vi "Client References Find Reference.vi"(2 "ID to Find (\"\")":string, 3 "TESTREFS (empty)":T1[](array[typedef])) -> (1 "Element":i32)   [LabVIEW 2011]
uses:
  Client References.ctl
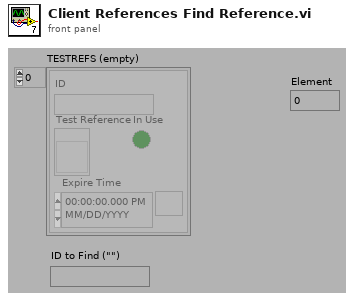
[diagram p1: front panel]
types:
  T1 = typedef "Client References.ctl" = cluster{"ID":string, "Test Reference":refnum<vi>, "In Use":bool, "Expire Time":timestamp}
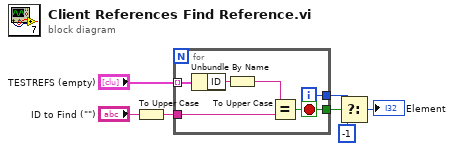
[diagram p0: block diagram]
diagram:
  n1 = To Upper Case(1:"ID to Find (\"\")") -> (0:w7:string)
  n2 = for {
    tunnel: "TESTREFS (empty)" -> [w13] mode=indexing
    tunnel: w7 -> [w12]
    tunnel: [w10] -> w4
    tunnel: [w9] -> w5
    i -> [w10]
    stop <- w9 stop-if-true
    n3 = Unbundle By Name(w13) -> ("ID"=w11:string)
    n4 = To Upper Case(1:w11) -> (0:w8:string)
    n5 = Equal?(x=w8, y=w12) -> (x = y?=w9:bool)
  }
  n6 = Select(t=w4, s=w5, f=-1) -> (s? t:f=→"Element":i32)
